vi "Configure DC Current5.vi"(8 "error in (no error)":errorcluster, 10 "measurementservice_SMUConfigRequest_Data":T3, 11 "SMUSession":refnum<k15>) -> (0 "error out":errorcluster, 2 "measurementservice_SMUConfigResponse_Data":T1)   [LabVIEW 2019, in "HVC5.lvlib" / "HVC5.lvclass"]
doc: "Demonstrates how to use the DC Current Output Function to force an output current. This example initializes a session, configures the Output Function, Sense, Autorange, Current Level and Voltage Limit, initiates generation, waits for a specified delay, and measures the voltage and current output. This example uses Single Point source mode."
uses:
  HVC5 Class/HVC5.lvclass
  HVC5 Class/RPC Messages/measurementservice_SMUConfigRequest/measurementservice_SMUConfigRequest_Data.ctl
  HVC5 Class/RPC Messages/measurementservice_SMUConfigResponse/measurementservice_SMUConfigResponse_Data.ctl
  HVC5 Class/RPC Messages/measurementservice_ErrorOut/measurementservice_ErrorOut_Data.ctl
panel:
  # "Overview: Demonstrates how to use the DC Current Output Function to force an output current.  \nThis example initializes a session, configures the Output Function, Sense, Autorange, Current Level \nand Voltage Limit, initiates generation, waits for a specified delay, and measures the voltage and \ncurrent output.  \nRequirements: NI-DCPower\nInstructions:\n1. Select the appropriate device in the Resource Name control.\n2. Configure the parameters of the DC Current signal you'd like to output.\n3. Run the VI."
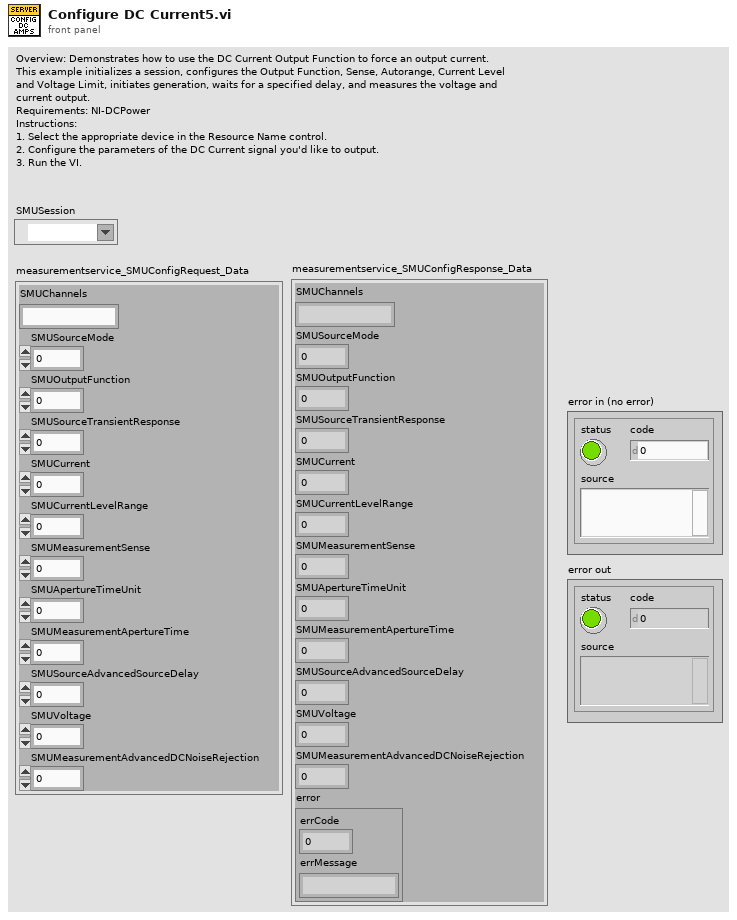
[diagram p1: front panel]
types:
  T1 = typedef "HVC5.lvlib/HVC5.lvclass/measurementservice_SMUConfigResponse_Data.ctl" = cluster{"SMUChannels":string, "SMUSourceMode":i32, "SMUOutputFunction":i32, "SMUSourceTransientResponse":i32, "SMUCurrent":sgl, "SMUCurrentLevelRange":sgl, "SMUMeasurementSense":i32, "SMUApertureTimeUnit":i32, "SMUMeasurementApertureTime":sgl, "SMUSourceAdvancedSourceDelay":sgl, "SMUVoltage":sgl, "SMUMeasurementAdvancedDCNoiseRejection":i32, "error":T2}
  T2 = typedef "HVC5.lvlib/HVC5.lvclass/measurementservice_ErrorOut_Data.ctl" = cluster{"errCode":i32, "errMessage":string}
  T3 = typedef "HVC5.lvlib/HVC5.lvclass/measurementservice_SMUConfigRequest_Data.ctl" = cluster{"SMUChannels":string, "SMUSourceMode":i32, "SMUOutputFunction":i32, "SMUSourceTransientResponse":i32, "SMUCurrent":sgl, "SMUCurrentLevelRange":sgl, "SMUMeasurementSense":i32, "SMUApertureTimeUnit":i32, "SMUMeasurementApertureTime":sgl, "SMUSourceAdvancedSourceDelay":sgl, "SMUVoltage":sgl, "SMUMeasurementAdvancedDCNoiseRejection":i32}
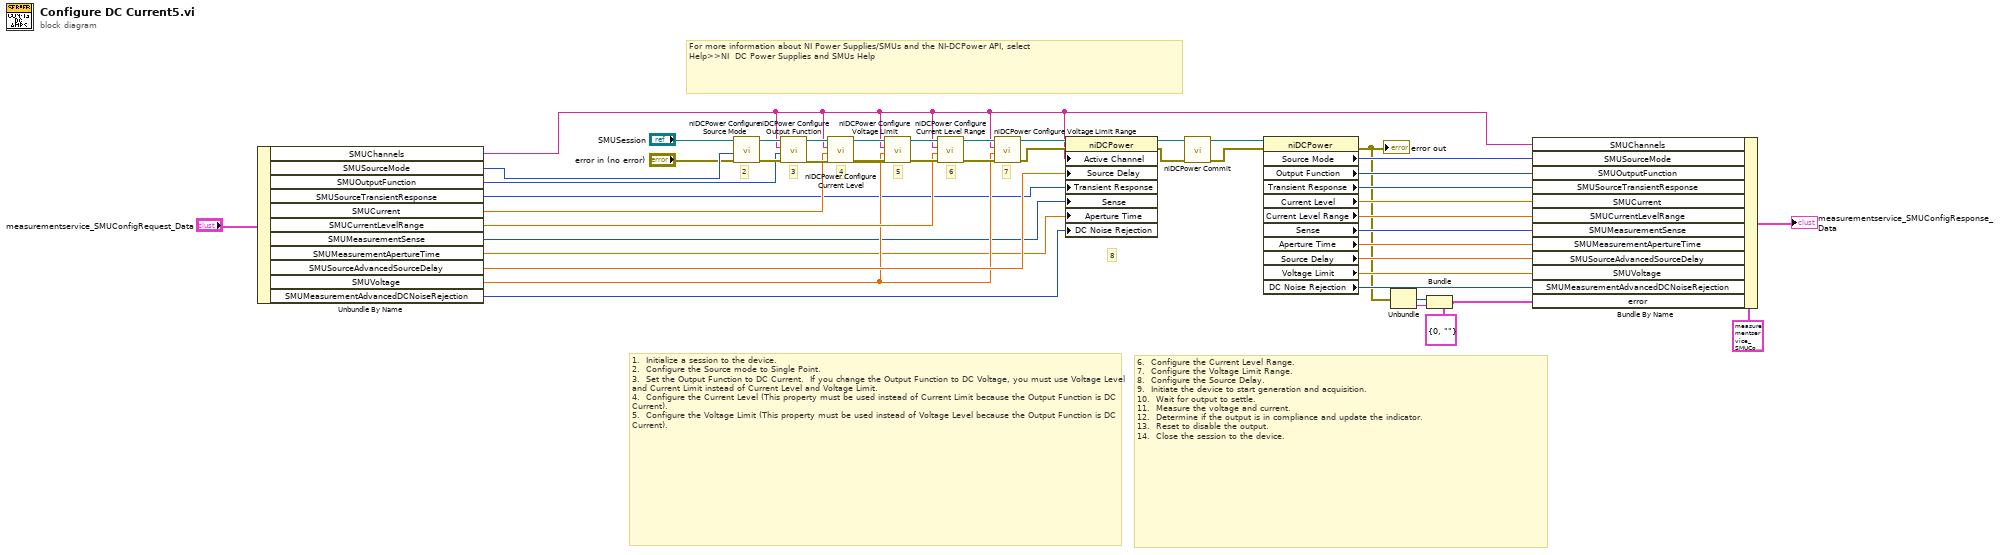
[diagram p0: block diagram]
diagram:
  # "For more information about NI Power Supplies/SMUs and the NI-DCPower API, select\nHelp>>NI  DC Power Supplies and SMUs Help"
  # "8"
  # "7"
  # "6"
  # "2"
  # "1.  Initialize a session to the device.\n2.  Configure the Source mode to Single Point.\n3.  Set the Output Function to DC Current.  If you change the Output Function to DC Voltage, you must use Voltage Level and Current Limit instead of Current Level and Voltage Limit.\n4.  Configure the Current Level (This property must be used instead of Current Limit because the Output Function is DC Current).\n5.  Configure the Voltage Limit (This property must be used instead of Voltage Level because the Output Function is DC Current)."
  # "3"
  # "6.  Configure the Current Level Range.\n7.  Configure the Voltage Limit Range.\n8.  Configure the Source Delay.\n9.  Initiate the device to start generation and acquisition.\n10.  Wait for output to settle.\n11.  Measure the voltage and current.\n12.  Determine if the output is in compliance and update the indicator.\n13.  Reset to disable the output.\n14.  Close the session to the device."
  # "5"
  # "4"
  n1 = Unbundle By Name("measurementservice_SMUConfigRequest_Data") -> ("SMUChannels"=w6:string, "SMUSourceMode"=w31:i32, "SMUOutputFunction"=w30:i32, "SMUSourceTransientResponse"=w25:i32, "SMUCurrent"=w29:sgl, "SMUCurrentLevelRange"=w28:sgl, "SMUMeasurementSense"=w24:i32, "SMUMeasurementApertureTime"=w23:sgl, "SMUSourceAdvancedSourceDelay"=w27:sgl, "SMUVoltage"=w26:sgl, "SMUMeasurementAdvancedDCNoiseRejection"=w22:i32)
  n2 = call <instrlib>:"niDCPower Configure Source Mode.vi"("error in (no error)"="error in (no error)", "source mode"=w31, "instrument handle"="SMUSession") -> ("error out"=w45:errorcluster, "instrument handle out"=w44:refnum<k15>)  [unwired: 7 out]
  n3 = call <instrlib>:"niDCPower Configure Output Function.vi"("error in (no error)"=w45, "output function"=w30, "channel name"=w6, "instrument handle"=w44) -> ("error out"=w37:errorcluster, "instrument handle out"=w36:refnum<k15>)  [unwired: 6 out]
  n4 = call <instrlib>:"niDCPower Configure Current Level.vi"("error in (no error)"=w37, "current level"=w29, "channel name"=w6, "instrument handle"=w36) -> ("error out"=w46:errorcluster, "instrument handle out"=w47:refnum<k15>)  [unwired: 6 out]
  n5 = call <instrlib>:"niDCPower Configure Voltage Limit.vi"("error in (no error)"=w46, "voltage limit"=w26, "channel name"=w6, "instrument handle"=w47) -> ("error out"=w43:errorcluster, "instrument handle out"=w42:refnum<k15>)  [unwired: 6 out]
  n6 = call <instrlib>:"niDCPower Configure Current Level Range.vi"("error in (no error)"=w43, "current level range"=w28, "channel name"=w6, "instrument handle"=w42) -> ("error out"=w41:errorcluster, "instrument handle out"=w40:refnum<k15>)  [unwired: 6 out]
  n7 = call <instrlib>:"niDCPower Configure Voltage Limit Range.vi"("error in (no error)"=w41, "voltage limit range"=w26, "channel name"=w6, "instrument handle"=w40) -> ("error out"=w38:errorcluster, "instrument handle out"=w39:refnum<k15>)  [unwired: 6 out]
  n8 = property class="niDCPower"(reference=w39, error in=w38, "Active Channel"=w6, "Source Delay"=w27, "Transient Response"=w25, "Sense"=w24, "Aperture Time"=w23, "DC Noise Rejection"=w22) -> (reference out=w35:refnum<k15>, error out=w34:errorcluster)
  n9 = call <instrlib>:"niDCPower Commit.vi"("error in (no error)"=w34, "instrument handle"=w35) -> ("error out"=w32:errorcluster, "instrument handle out"=w33:refnum<k15>)  [unwired: 8 in]
  n10 = property class="niDCPower"(reference=w33, error in=w32) -> (error out=w5:errorcluster, "Source Mode"=w21:i32, "Output Function"=w20:i32, "Transient Response"=w19:i32, "Current Level"=w18:dbl, "Current Level Range"=w17:dbl, "Sense"=w16:i32, "Aperture Time"=w15:dbl, "Source Delay"=w14:dbl, "Voltage Limit"=w13:dbl, "DC Noise Rejection"=w12:i32)  [unwired: 1 out]
  "error out" <- w5
  n11 = Unbundle(w5) -> ("code"=w3:i32, "source"=w2:string)  [unwired: 1 out]
  n12 = Bundle(cluster=T2 {"errCode"=0, "errMessage"=""} ("error"), "errCode"=w3, "errMessage"=w2) -> (w1:T2)
  n13 = Bundle By Name(cluster=T1 {"SMUChannels"="", "SMUSourceMode"=0, "SMUOutputFunction"=0, "SMUSourceTransientResponse"=0, "SMUCurrent"=0.0, "SMUCurrentLevelRange"=0.0, "SMUMeasurementSense"=0, "SMUApertureTimeUnit"=0, "SMUMeasurementApertureTime"=0.0, "SMUSourceAdvancedSourceDelay"=0.0, "SMUVoltage"=0.0, "SMUMeasurementAdvancedDCNoiseRejection"=0, "error"={"errCode"=0, "errMessage"=""}} ("measurementservice_SMUConfigResponse_Data"), "SMUChannels"=w6, "SMUSourceMode"=w21, "SMUOutputFunction"=w20, "SMUSourceTransientResponse"=w19, "SMUCurrent"=w18, "SMUCurrentLevelRange"=w17, "SMUMeasurementSense"=w16, "SMUMeasurementApertureTime"=w15, "SMUSourceAdvancedSourceDelay"=w14, "SMUVoltage"=w13, "SMUMeasurementAdvancedDCNoiseRejection"=w12, "error"=w1) -> (→"measurementservice_SMUConfigResponse_Data":T1)
